vi "Final.vi"() -> ()   [LabVIEW 2025]
uses:
  <vilib>/Analysis/baseanly.llb/Mean (DBL).vi
  <vilib>/Analysis/3filter.llb/Butterworth Filter (DBL).vi
  <vilib>/Analysis/NI_AALBase.lvlib
panel:
  out "Door":bool
  in  "Paitent Thermometer":dbl(slide) scale=30.0..42.0
  in  "Stress Level":dbl(slide) scale=0.0..100.0
  out "GSR Signal":dbl[](graph)
  out "GSR Level":string
  out "Skin Conductance (µS)":dbl
  in  "GSR STOP":bool
  out "ECG Waveform":dynamicdata(graph)
  out "Heart Rate (BPM)":dbl format="%#_2g"
  in  "Nurse Call Button":bool
  in  "Nurse Reset":bool
  out "NURSE ALERT":bool
  out "BPM Warning":bool
  out "Heart Status":string
  out "Temperature Warning":bool
  out "Temperature Statue":string
  out "Green (Patient Normal Or Relaxation Mode)\nRed (Patient is Stressed)":bool
  out "Fever":bool
  out "Normal Temp":bool
  out "Cold":bool
  out "Paient Temperature":dbl
  out "BMI":dbl
  out "BMR":dbl
  in  "Weight (Kg)":dbl
  in  "Height (cm)":dbl
  in  "Age (Years)":dbl
  in  "Gender":enum16{"Male", "Female"}(ring)
  in  "Thermometer":dbl(slide) scale=0.0..100.0
  in  "Temperture Control":dbl
  in  "CO2 Tank":dbl(slide) scale=0.0..100.0
  in  "smoke detector":dbl(slide) scale=0.0..100.0
  out "valve of CO2":bool
  in  "no one inside":bool
  in  "smoke set point":dbl(slide) scale=0.0..100.0
  out "alarm":bool
  in  "Mode":enum16{"Auto", "Manual Warm", "Manual Cool"}(ring)
  in  "Fan":enum16{"High", "Mid", "Low"}(ring)
  in  "stop":bool
  out "?":dbl
  # "Monitors"
  # "Nurse  Dashboard"
  # "Paient Dashboard"
  # "Stress Monitor"
  # "Temperature Monitors"
  # "Firestop Control Unit"
  # "Room Temperature Control Unit"
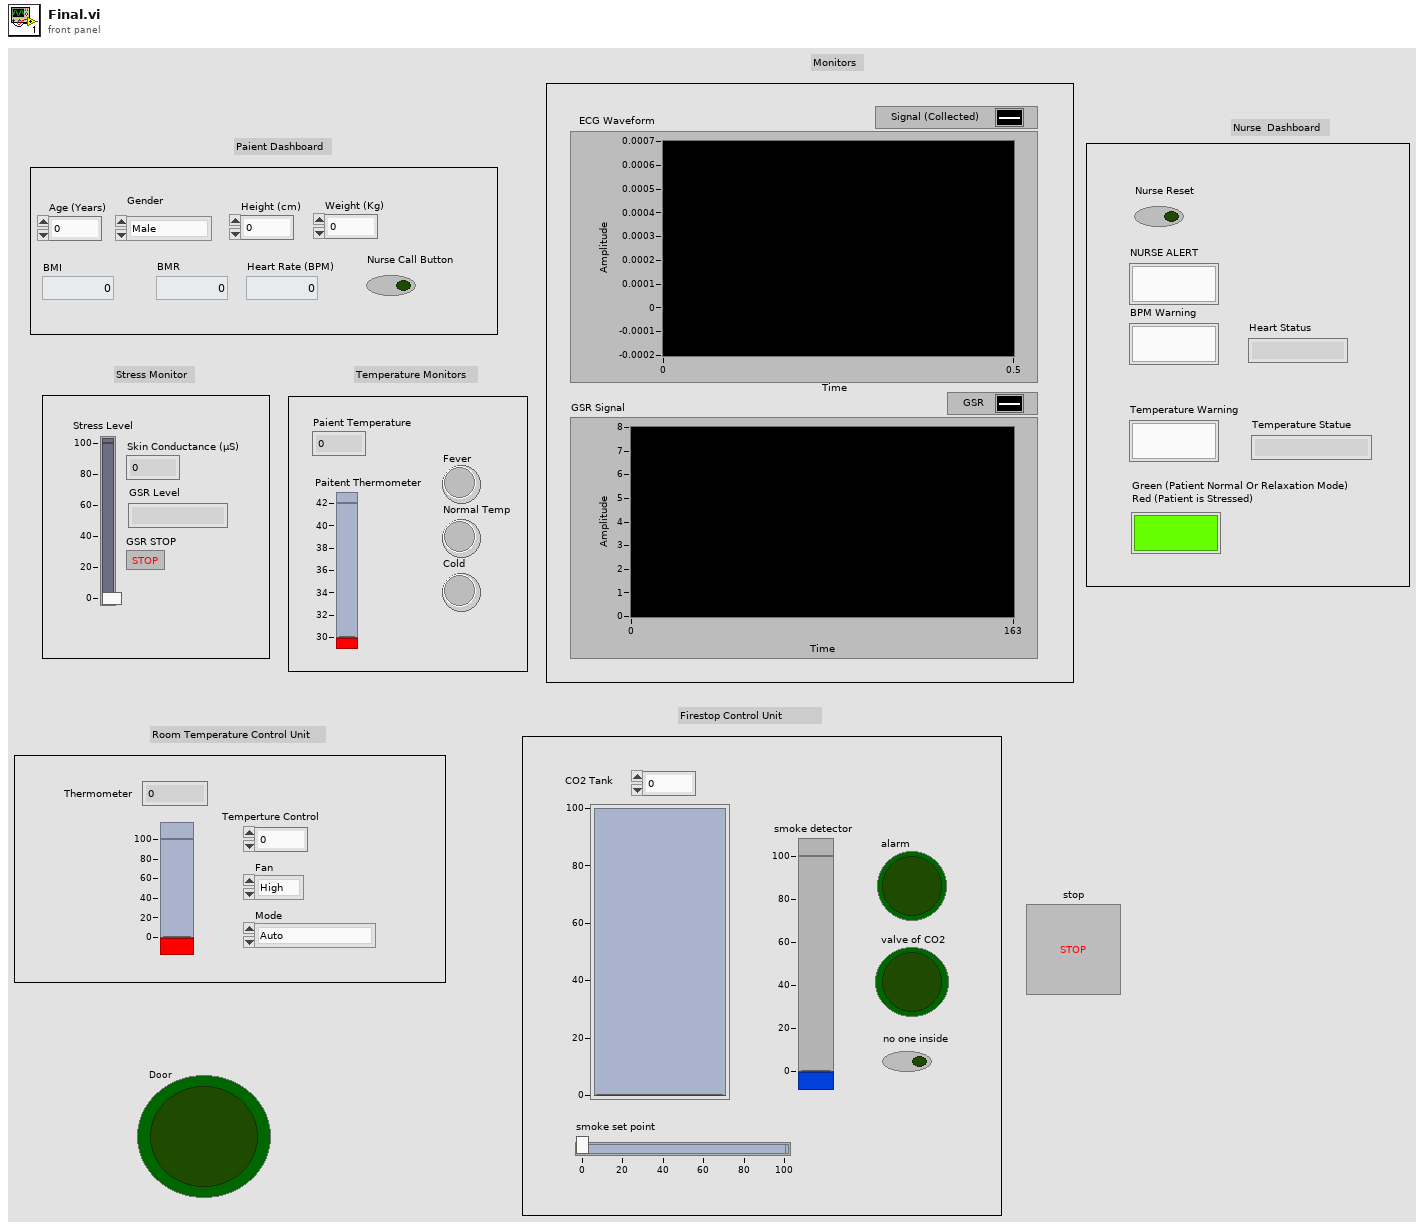
[diagram p1: front panel]
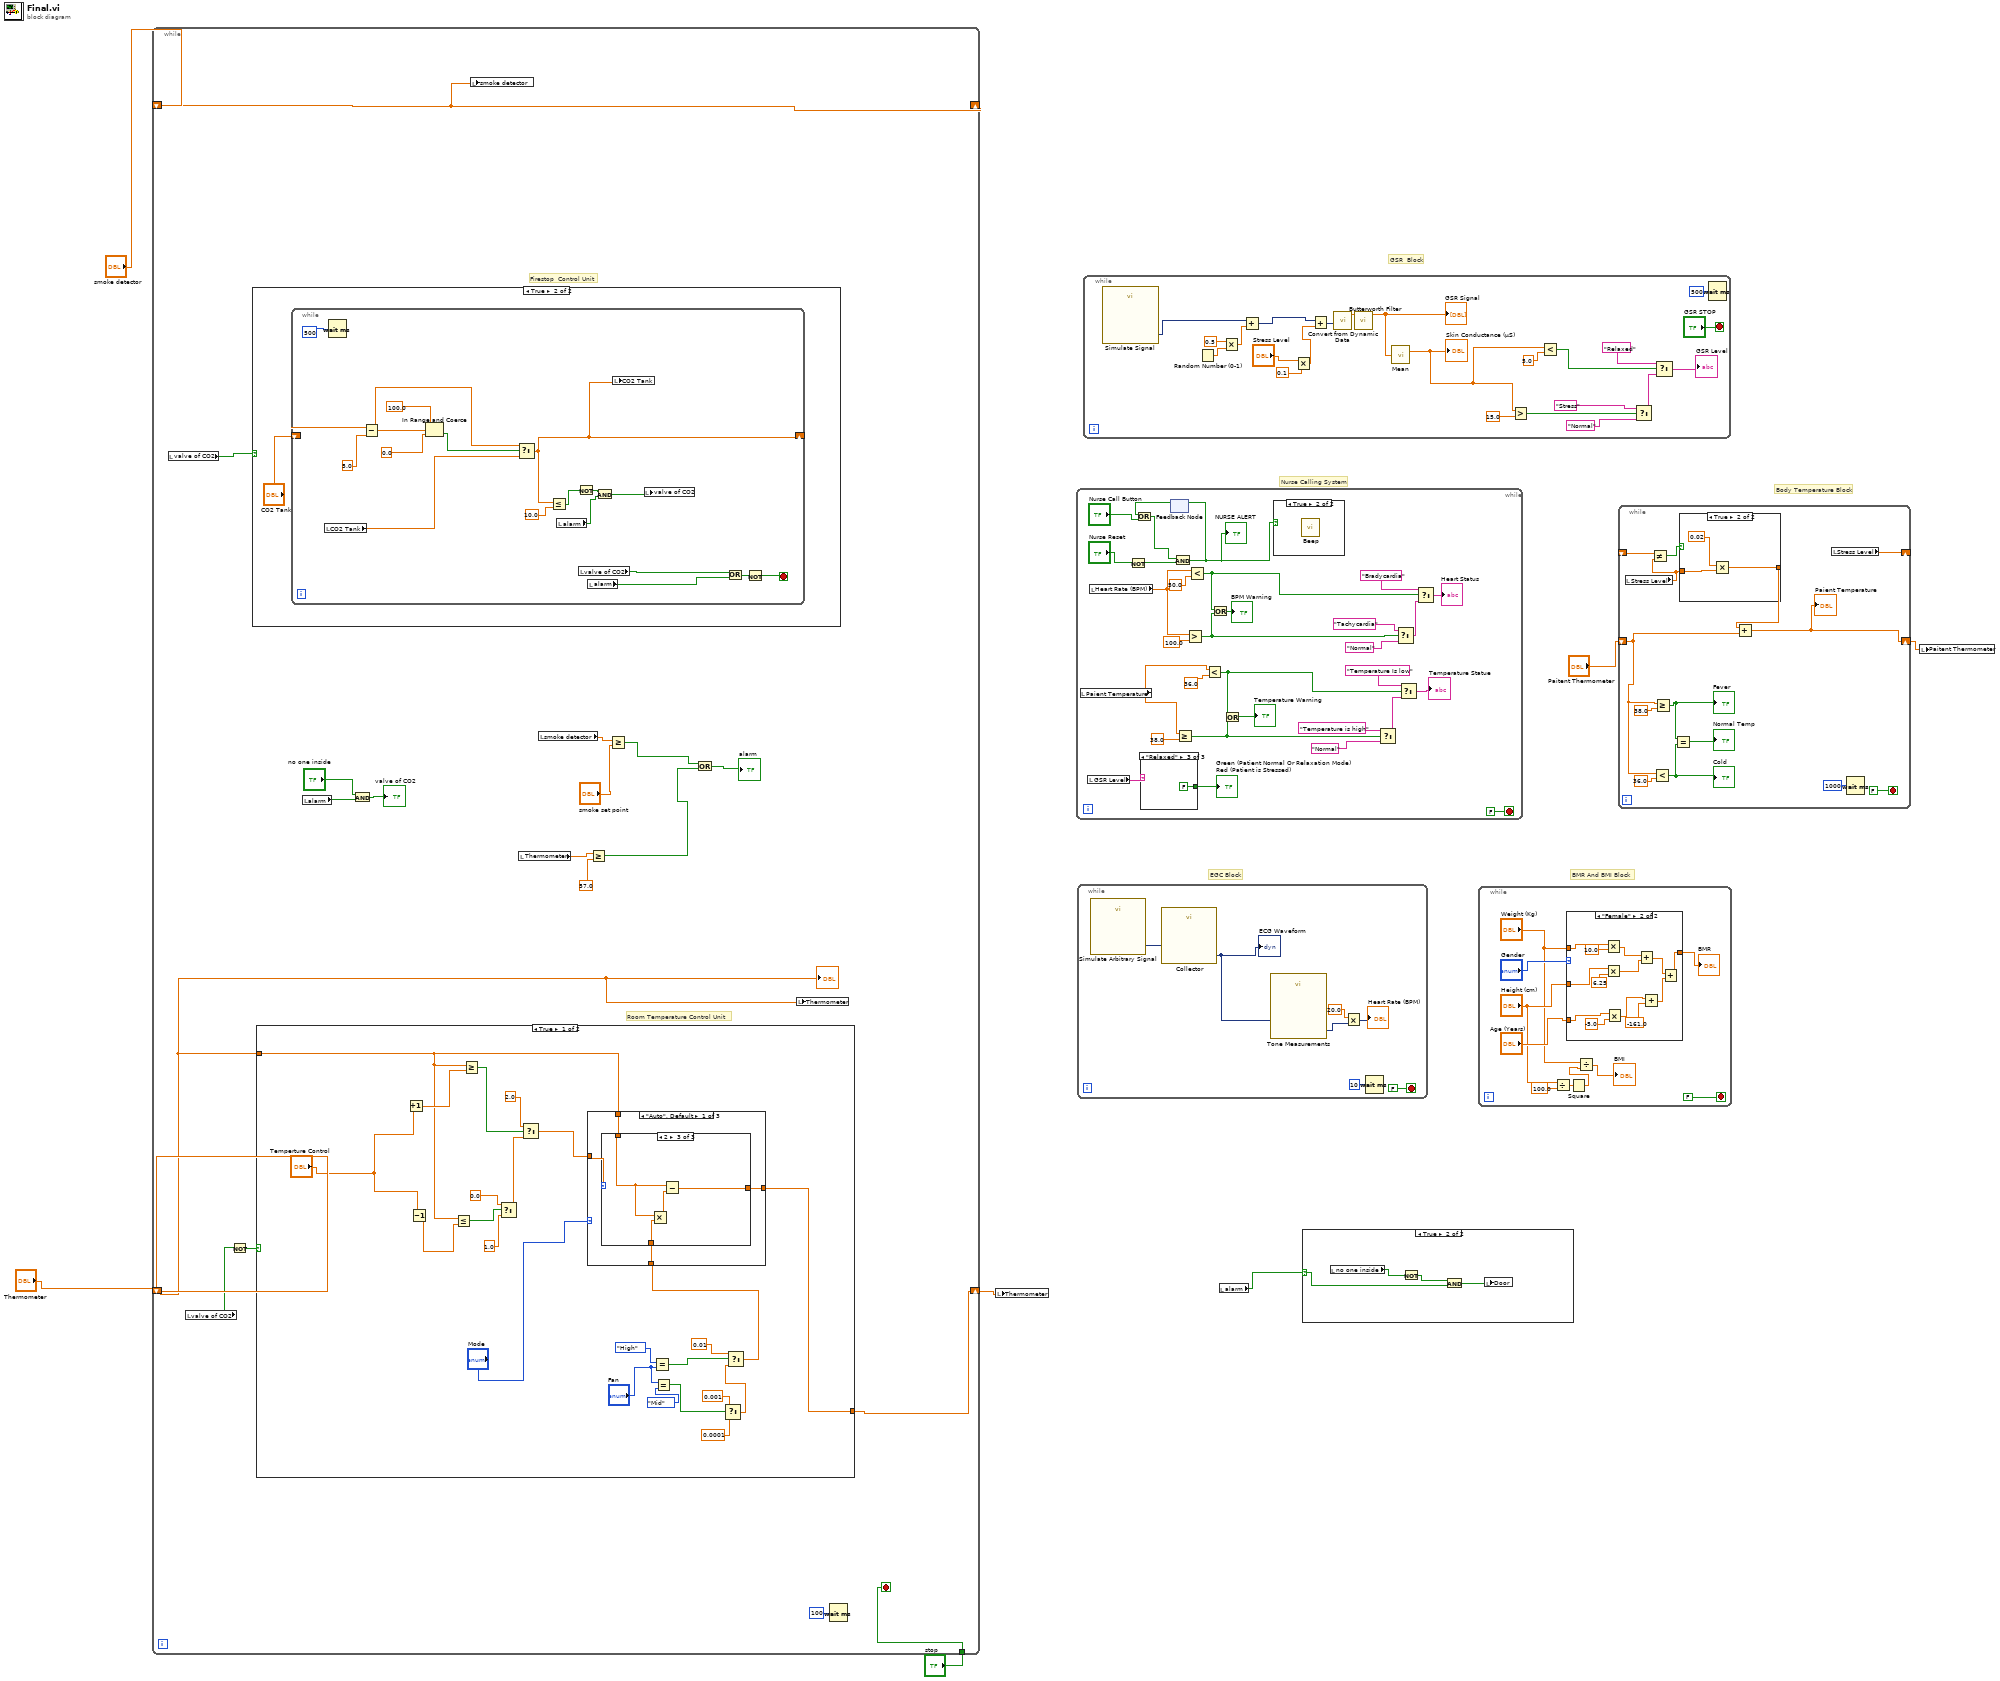
[diagram p0: block diagram]
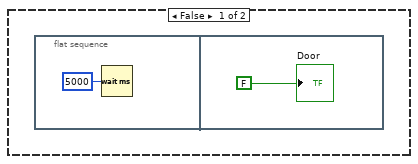
[diagram p2: hidden frame]
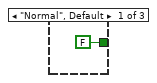
[diagram p3: hidden frame]
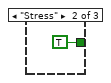
[diagram p4: hidden frame]
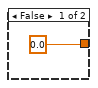
[diagram p6: hidden frame]
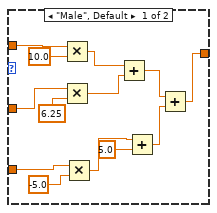
[diagram p7: hidden frame]
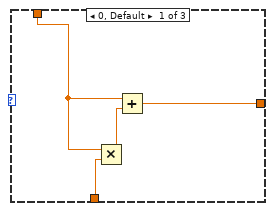
[diagram p9: hidden frame]
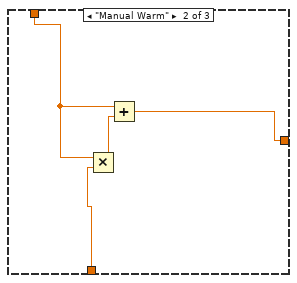
[diagram p11: hidden frame]
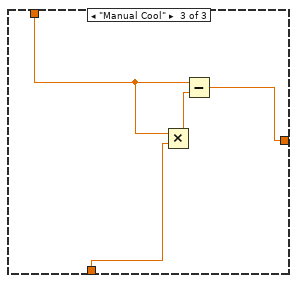
[diagram p12: hidden frame]
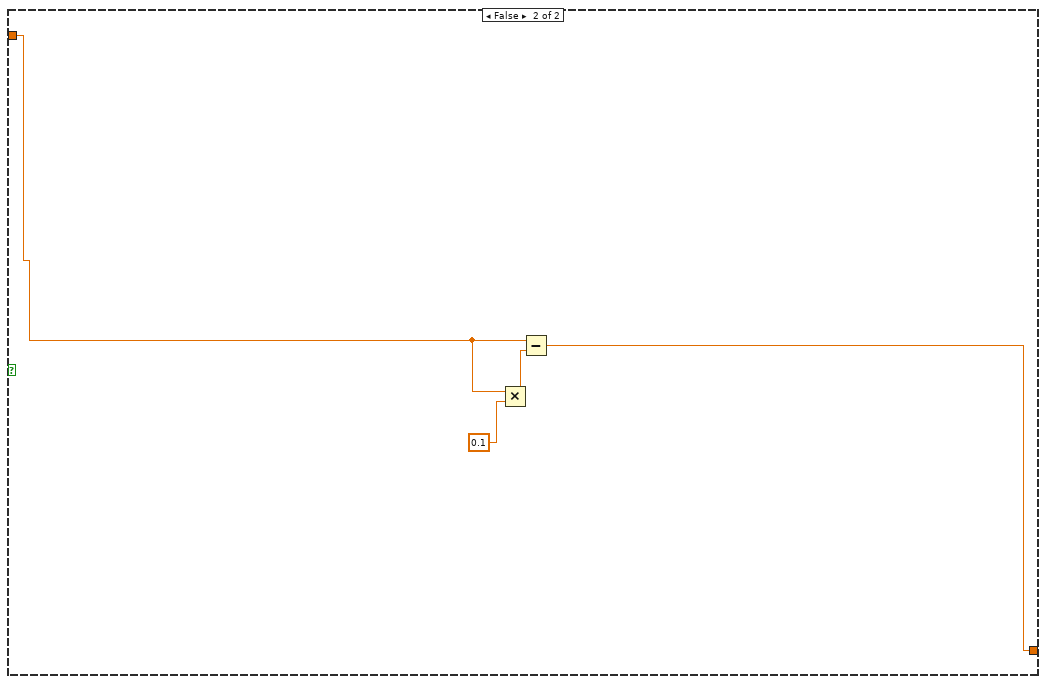
[diagram p13: hidden frame]
diagram:
  # "EGC Block"
  # "Nurse Calling System"
  # "Body Temperature Block"
  # "BMR And BMI Block"
  # "GSR  Block"
  n1 = while {
    tunnel: "stop" -> [w25]
    shift-right: [w24] -> w4
    shift-left: "Thermometer" -> [w10]
    shift-right: [w13] -> _
    shift-left: "smoke detector" -> [w13]
    stop <- w25 stop-if-true
    # "Room Temperature Control Unit"
    # "Firestop  Control Unit"
    n2 = local read "valve of CO2"() -> (w11:bool)
    n3 = local read "valve of CO2"() -> (w14:bool)
    n4 = Not(x=w14) -> (.not. x?=w17:bool)
    n5 = case shown="True" w11 {
      frame False {
      }
      frame True {
        n6 = while {
          shift-right: [w33] -> _
          shift-left: "CO2 Tank" -> [w44]
          stop <- w27 stop-if-true
          n7 = local read "CO2 Tank"() -> (w32:dbl)
          n8 = Wait (ms)(milliseconds to wait=u32 500) -> ()  [unwired: 1 out]
          n9 = Subtract(x=w44, y=5.0) -> (x-y=w38:dbl)
          n10 = In Range and Coerce(upper limit=100.0, x=w38, lower limit=0.0 ("x")) -> (In Range?=w39:bool)  [unwired: 1 out]
          n11 = Select(t=w38, s=w39, f=w32) -> (s? t:f=w33:dbl)
          n12 = Less Or Equal?(x=w33, y=10.0) -> (x <= y?=w31:bool)
          n13 = local read "alarm"() -> (w28:bool)
          n14 = Not(x=w31) -> (.not. x?=w30:bool)
          n15 = local read "valve of CO2"() -> (w34:bool)
          n16 = local read "alarm"() -> (w37:bool)
          n17 = And(x=w30, y=w28) -> (x .and. y?=w29:bool)
          n18 = local write "CO2 Tank"(w33) -> ()
          n19 = local write "valve of CO2"(w29) -> ()
          n20 = Or(x=w34, y=w37) -> (x .or. y?=w36:bool)
          n21 = Not(x=w36) -> (.not. x?=w27:bool)
        }
      }
    }
    n22 = case shown="True" w17 {
      tunnel: [w47 w89] -> w24
      tunnel: w10 -> [w46 w90]
      frame True {
        n23 = Increment(x="Temperture Control") -> (x+1=w67:dbl)
        n24 = Decrement(x="Temperture Control") -> (x-1=w66:dbl)
        n25 = Less Or Equal?(x=w46, y=w66) -> (x <= y?=w64:bool)
        n26 = Greater Or Equal?(x=w46, y=w67) -> (x >= y?=w65:bool)
        n27 = Select(t=0.0, s=w64, f=1.0) -> (s? t:f=w62:dbl)
        n28 = Select(t=2.0, s=w65, f=w62) -> (s? t:f=w63:dbl)
        n29 = Equal?(x=enum16{"High", "Mid", "Low"}."High", y="Fan") -> (x = y?=w55:bool)
        n30 = Equal?(x="Fan", y=enum16{"High", "Mid", "Low"}."Mid") -> (x = y?=w58:bool)
        n31 = Select(t=0.001, s=w58, f=0.0001) -> (s? t:f=w57:dbl)
        n32 = Select(t=0.01, s=w55, f=w57) -> (s? t:f=w49:dbl)
        n33 = case shown="\"Auto\", Default" "Mode" {
          tunnel: w63 -> [w71 _ _]
          tunnel: w46 -> [w70 w83 w87]
          tunnel: [w69 w81 w85] -> w47
          tunnel: w49 -> [w68 w82 w86]
          frame "Auto", Default {
            n34 = case shown="2" w71 {
              tunnel: w70 -> [w73 w76 w79]
              tunnel: [w72 w76 w80] -> w69
              tunnel: w68 -> [w74 _ w77]
              frame 0, Default {
                n35 = Multiply(x=w73, y=w74) -> (x*y=w75:dbl)
                n36 = Add(x=w73, y=w75) -> (x+y=w72:dbl)
              }
              frame 1 {
              }
              frame 2 {
                n37 = Multiply(x=w79, y=w77) -> (x*y=w78:dbl)
                n38 = Subtract(x=w79, y=w78) -> (x-y=w80:dbl)
              }
            }
          }
          frame "Manual Warm" {
            n39 = Multiply(x=w83, y=w82) -> (x*y=w84:dbl)
            n40 = Add(x=w83, y=w84) -> (x+y=w81:dbl)
          }
          frame "Manual Cool" {
            n41 = Multiply(x=w87, y=w86) -> (x*y=w88:dbl)
            n42 = Subtract(x=w87, y=w88) -> (x-y=w85:dbl)
          }
        }
      }
      frame False {
        n43 = Multiply(x=w90, y=0.1) -> (x*y=w91:dbl)
        n44 = Subtract(x=w90, y=w91) -> (x-y=w89:dbl)
      }
    }
    n45 = local read "alarm"() -> (w16:bool)
    n46 = And(x="no one inside", y=w16) -> (x .and. y?=→"valve of CO2":bool)
    n47 = local write "smoke detector"(w13) -> ()
    n48 = local read "Thermometer"() -> (w9:dbl)
    n49 = local read "smoke detector"() -> (w8:dbl)
    n50 = Greater Or Equal?(x=w9, y=57.0 ("x")) -> (x >= y?=w18:bool)
    n51 = Greater Or Equal?(x=w8, y="smoke set point") -> (x >= y?=w19:bool)
    n52 = Or(x=w19, y=w18) -> (x .or. y?=→"alarm":bool)
    n53 = local write "Thermometer"(w10) -> ()
    n54 = Wait (ms)(milliseconds to wait=u32 100) -> ()  [unwired: 1 out]
    "?" <- w10
  }
  n55 = local write "Thermometer"(w4) -> ()
  n56 = while {
    stop <- FALSE stop-if-true
    n57 = local read "Paient Temperature"() -> (w99:dbl)
    n58 = local read "GSR Level"() -> (w96:string)
    n59 = local read "Heart Rate (BPM)"() -> (w118:dbl)
    n60 = Not(x="Nurse Reset") -> (.not. x?=w122:bool)
    n61 = case shown="\"Relaxed\"" w96 {
      tunnel: [FALSE ("Green (Patient Normal Mode)\nRed (Patient is Stressed)") TRUE ("Green (Patient Normal Mode)\nRed (Patient is Stressed)") FALSE ("Green (Patient Normal Mode)\nRed (Patient is Stressed)")] -> w95
      frame "Normal", Default {
      }
      frame "Stress" {
      }
      frame "Relaxed" {
      }
    }
    "Green (Patient Normal Or Relaxation Mode)\nRed (Patient is Stressed)" <- w95
    n62 = feedback #1() -> (w93:bool)  [unwired: 1 in]
    n63 = Or(x=w93, y="Nurse Call Button") -> (x .or. y?=w121:bool)
    n64 = And(x=w121, y=w122) -> (x .and. y?=w120:bool)
    "NURSE ALERT" <- w120
    n65 = feedback-in #1(w120) -> ()
    n66 = Greater Or Equal?(x=w99, y=38.0) -> (x >= y?=w97:bool)
    n67 = Greater?(x=w118, y=100.0) -> (0:w100:bool)
    n68 = Less?(x=w118, y=50.0) -> (x < y?=w101:bool)
    n69 = Less?(x=w99, y=36.0) -> (x < y?=w98:bool)
    n70 = Or(x=w101, y=w100) -> (x .or. y?=→"BPM Warning":bool)
    n71 = Or(x=w98, y=w97) -> (x .or. y?=→"Temperature Warning":bool)
    n72 = case shown="True" w120 {
      frame False {
      }
      frame True {
        n73 = call <vilib>:"Beep.vi"() -> ()  [unwired: 12 in]
      }
    }
    n74 = Select(t="Temperature is high", s=w97, f="Normal") -> (s? t:f=w103:string)
    n75 = Select(t="Tachycardia", s=w100, f="Normal") -> (s? t:f=w110:string)
    n76 = Select(t="Temperature Is low", s=w98, f=w103) -> (s? t:f=→"Temperature Statue":string)
    n77 = Select(t="Bradycardia", s=w101, f=w110) -> (s? t:f=→"Heart Status":string)
  }
  n78 = while {
    stop <- FALSE stop-if-true
    n79 = call "Simulate Arbitrary Signal"() -> ("Signal"=w130:dynamicdata)  [unwired: 9 in, 2 out]
    n80 = call "Collector"("Signals"=w130) -> ("Collected Signals"=w133:dynamicdata)  [unwired: 9 in, 1 out]
    "ECG Waveform" <- w133
    n81 = call "Tone Measurements"("Signals"=w133) -> ("Frequency"=w129:dynamicdata)  [unwired: 9 in, 1 out]
    n82 = Multiply(x=20.0, y=w129) -> (x*y=→"Heart Rate (BPM)":dynamicdata)
    n83 = Wait (ms)(milliseconds to wait=u32 10) -> ()  [unwired: 1 out]
  }
  n84 = while {
    stop <- "GSR STOP" stop-if-true
    n85 = call "Simulate Signal"() -> ("Sine"=w154:dynamicdata)  [unwired: 14 in, 1 out]
    n86 = Random Number (0-1)() -> (number: 0 to 1=w156:dbl)
    n87 = Multiply(x=0.5, y=w156) -> (x*y=w153:dbl)
    n88 = Add(x=w154, y=w153) -> (x+y=w150:dynamicdata)
    n89 = Multiply(x="Stress Level", y=0.1) -> (x*y=w149:dbl)
    n90 = Add(x=w150, y=w149) -> (x+y=w148:dynamicdata)
    n91 = call "Convert from Dynamic Data"("Dynamic Data Type"=w148) -> ("Array"=w147:dbl[])  [unwired: 3 in]
    n92 = call-poly <vilib>:"Butterworth Filter.vi"("X"=w147) -> ("Filtered X"=w146:dbl[])  [unwired: 7 in, 1 out]
    "GSR Signal" <- w146
    n93 = call-poly <vilib>:"Mean.vi"("X"=w146) -> ("mean"=w136:dbl)  [unwired: 1 out]
    "Skin Conductance (µS)" <- w136
    n94 = Greater?(x=w136, y=15.0) -> (0:w145:bool)
    n95 = Less?(x=w136, y=5.0) -> (x < y?=w144:bool)
    n96 = Select(t="Stress", s=w145, f="Normal") -> (s? t:f=w143:string)
    n97 = Select(t="Relaxed", s=w144, f=w143) -> (s? t:f=→"GSR Level":string)
    n98 = Wait (ms)(milliseconds to wait=u32 500) -> ()  [unwired: 1 out]
  }
  n99 = local read "alarm"() -> (w1:bool)
  n100 = case shown="True" w1 {
    selector: w1 -> [_ w160]
    frame False {
      n101 = flat-sequence {
        frame #0 {
          n102 = Wait (ms)(milliseconds to wait=u32 5000) -> ()  [unwired: 1 out]
        }
        frame #1 {
          "Door" <- FALSE
        }
      }
    }
    frame True {
      n103 = local read "no one inside"() -> (w162:bool)
      n104 = Not(x=w162) -> (.not. x?=w161:bool)
      n105 = And(x=w161, y=w160) -> (x .and. y?=w159:bool)
      n106 = local write "Door"(w159) -> ()
    }
  }
  n107 = while {
    stop <- FALSE stop-if-true
    n108 = Divide(x="Height (cm)", y=100.0) -> (x/y=w164:dbl)
    n109 = case shown="\"Female\"" "Gender" {
      tunnel: "Weight (Kg)" -> [w185 w189]
      tunnel: "Height (cm)" -> [w183 w188]
      tunnel: "Age (Years)" -> [w181 w187]
      tunnel: [w173 w186] -> w170
      frame "Male", Default {
        n110 = Multiply(x=w185, y=10.0) -> (x*y=w179:dbl)
        n111 = Multiply(x=w183, y=6.25) -> (x*y=w178:dbl)
        n112 = Multiply(x=w181, y=-5.0) -> (x*y=w177:dbl)
        n113 = Add(x=w179, y=w178) -> (x+y=w175:dbl)
        n114 = Add(x=w177, y=5.0) -> (x+y=w174:dbl)
        n115 = Add(x=w175, y=w174) -> (x+y=w173:dbl)
      }
      frame "Female" {
        n116 = Multiply(x=w189, y=10.0) -> (x*y=w195:dbl)
        n117 = Multiply(x=w188, y=6.25) -> (x*y=w194:dbl)
        n118 = Multiply(x=w187, y=-5.0) -> (x*y=w193:dbl)
        n119 = Add(x=w195, y=w194) -> (x+y=w191:dbl)
        n120 = Add(x=w193, y=-161.0) -> (x+y=w190:dbl)
        n121 = Add(x=w191, y=w190) -> (x+y=w186:dbl)
      }
    }
    "BMR" <- w170
    n122 = Square(x=w164) -> (x^2=w163:dbl)
    n123 = Divide(x="Weight (Kg)", y=w163) -> (x/y=→"BMI":dbl)
  }
  n124 = while {
    shift-right: [w204] -> w2
    shift-left: "Paitent Thermometer" -> [w205]
    shift-right: [w201] -> _
    shift-left: _ -> [w202]
    stop <- FALSE stop-if-true
    n125 = local read "Stress Level"() -> (w200:dbl)
    n126 = Not Equal?(x=w202, y=w200) -> (x != y?=w199:bool)
    n127 = Less?(x=w205, y=36.0) -> (x < y?=w207:bool)
    "Cold" <- w207
    n128 = Greater Or Equal?(x=w205, y=38.0) -> (x >= y?=w208:bool)
    "Fever" <- w208
    n129 = Equal?(x=w208, y=w207) -> (x = y?=→"Normal Temp":bool)
    n130 = case shown="True" w199 {
      tunnel: [0.0 w214] -> w203
      tunnel: w200 -> [_ w215]
      frame False {
      }
      frame True {
        n131 = Multiply(x=0.02, y=w215) -> (x*y=w214:dbl)
      }
    }
    n132 = Add(x=w203, y=w205) -> (x+y=w204:dbl)
    "Paient Temperature" <- w204
    n133 = local read "Stress Level"() -> (w201:dbl)
    n134 = Wait (ms)(milliseconds to wait=u32 1000) -> ()  [unwired: 1 out]
  }
  n135 = local write "Paitent Thermometer"(w2) -> ()
